vi "FocusedImageWithTrigOut.vi"() -> ()   [LabVIEW 2015]
panel:
  in  "quit remote":bool
  in  "stop sequence":bool
  in  "start sequence":bool
  in  "load sequence":bool
  in  "stop":bool
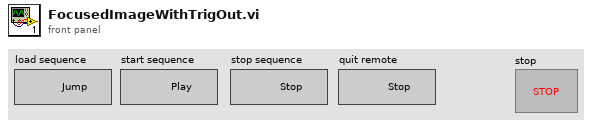
[diagram p1: front panel]
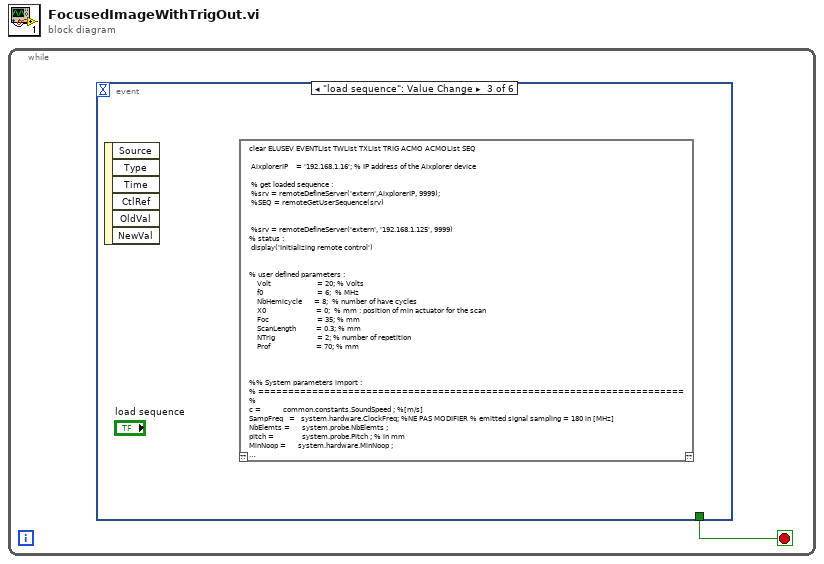
[diagram p0: block diagram]
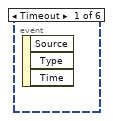
[diagram p2: hidden frame]
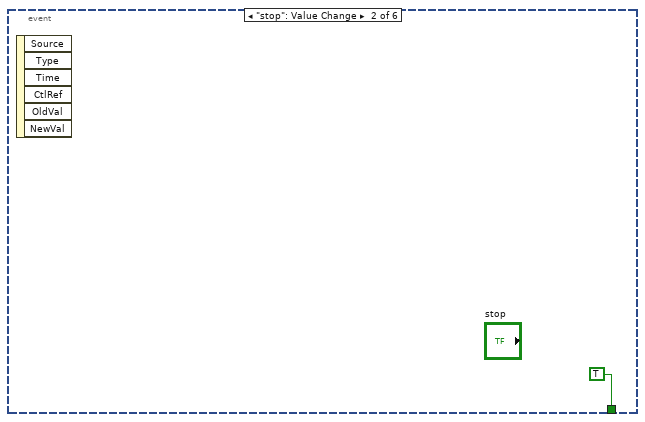
[diagram p3: hidden frame]
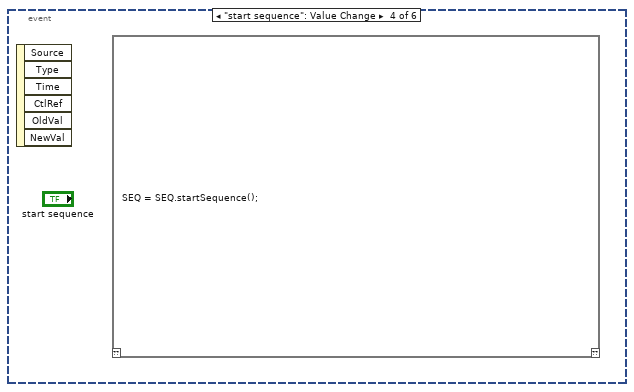
[diagram p4: hidden frame]
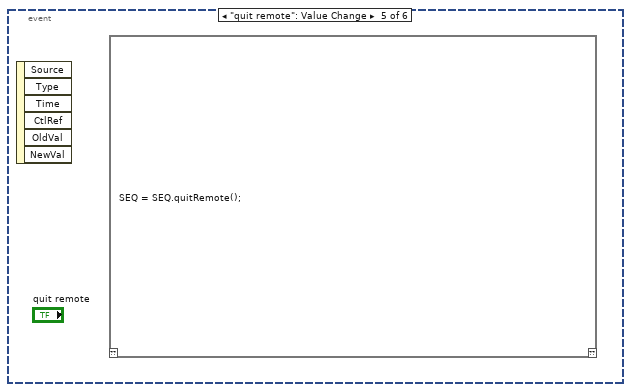
[diagram p5: hidden frame]
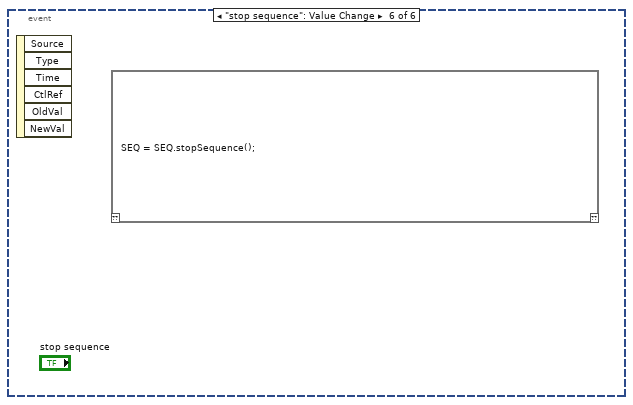
[diagram p6: hidden frame]
diagram:
  n1 = while {
    stop <- w1 stop-if-true
    n2 = event shown="[2] \"load sequence\": Value Change" {
      selector: _ -> [_ _ _ _ _ _]
      dyn-events: _ -> [_ _ _ _ _ _]
      timeout: _ -> [_ _ _ _ _ _]
      tunnel: [_ TRUE _ _ _ _] -> w1
      event Timeout {
        n3 = event-data() -> ()  [unwired: 1 in, 3 out]
      }
      event "stop": Value Change {
        n4 = event-data() -> ()  [unwired: 1 in, 6 out]
      }
      event "load sequence": Value Change {
        n5 = event-data() -> ()  [unwired: 1 in, 6 out]
        n6 = script code="clear ELUSEV EVENTList TWList TXList TRIG ACMO ACMOList SEQ\n\n AixplorerIP    = '192.168.1.16'; % IP address of the Aixplorer device\n \n % get loaded sequence :\n %srv = remoteDefineServer('extern',AixplorerIP, 9999);\n %SEQ = remoteGetUserSequence(srv)\n \n \n %srv = remoteDefineServer('extern', '192.168.1.125', 9999)\n% status :\n display('Initializing remote control')\n\n\n% user defined parameters :\n    Volt                       = 20; % Volts\n    f0                           = 6;  % MHz\n    NbHemicycle      = 8;  % number of have cycles\n    X0                         = 0;  % mm : position of min actuator for the scan\n    Foc                        = 35; % mm\n    ScanLength          = 0.3; % mm\n    NTrig                     = 2; % number of repetition\n    Prof                       = 70; % mm\n\n\n\n%% System parameters import :\n% ======================================================================= %\nc =           common.constants.SoundSpeed ; %[m/s]\nSampFreq   =   system.hardware.ClockFreq; %NE PAS MODIFIER % emitted signal sampling = 180 in [MHz]\nNbElemts =      system.probe.NbElemts ; \npitch =              system.probe.Pitch ; % in mm\nMinNoop =      system.hardware.MinNoop ;\n\n%% Focusing parameters\n% ======================================================================= %\nTxWidth       = Foc/2;           % mm : effective width for focus line\nPropagationTime = (Prof)/(c)*1e3 ; % duration for one line in \\mu s\n\n\nNoOp       = 500;             % µs minimum time between two US pulses, (5 by default ??)\nFIRBandwidth = 90;            % FIR receiving bandwidth [%] - center frequency = UF.TwFreq\nRxFreq    = 6;                % Receiving center frequency MHz , ??\n\nTrigOut    = ceil(PropagationTime);  % µs\nPause      = max( NoOp - ceil(PropagationTime) , MinNoop ); % pause duration in µs\n\n% ======================================================================= %\n%% Codage en arbitrary : delay matrix and waveform\ndt_s = 1/(SampFreq);      % unit us\npulseDuration = NbHemicycle*(0.5/f0) ; % US inital pulse duration in us\n\n\n%% Delay Law [us]\n% ======================================================================= %\n% c[m/s] -> [mm/us] ; eg factor 1e-3 in the above expression\nDelay = sqrt(Foc^2+(TxWidth/2)^2)/(c*1e-3) ...\n        - 1/(c*1e-3)*sqrt(Foc^2+((0:pitch:TxWidth)-TxWidth/2).^2);\n     \n%   figure;\n%   plot(Delay,'r')\n%   xlabel('actuator')\n%   ylabel('delays (\\mu s)')\n\n% number of steps offset dt_s for each actuators position : \n DlySmpl = round(Delay/dt_s); \n\n % common waveform for emission, square envoppe - non apodized:\n T_Wf = 0:dt_s:0.5*NbHemicycle/f0;\n Wf = sin(2*pi*f0*T_Wf); \n \n % number of time-points necessary = points in waveform + maximum delay\n % offset\n N_T = length(Wf) + max(DlySmpl); \n\n%%% construction of a delay matrix : one column / actuator\n WF_mat = zeros(N_T,length(Delay));\n\n for j = 1:length(Delay)\n     % offset for each actuator + normal waveform init\n     WF_mat(DlySmpl(j)+(1:length(Wf)),j) = Wf;\n end\n \n WF_mat_sign = sign(WF_mat); % l'aixplorer code sur 3 niveaux [-1,0,1]\n\n% figure(470);\n% imagesc((0:pitch:TxWidth)-TxWidth/2,1:N_T, WF_mat);\n% grid on\n% title('input waveform');\n% xlabel('position x');\n% ylabel('offset num ??');\n\n% ======================================================================= %\n%% Arbitrary definition of US events\n% \n% % Elusev\n\n% \n FC = remote.fc('Bandwidth', FIRBandwidth , 0);\n RX = remote.rx('fcId', 1, 'RxFreq', RxFreq, 'QFilter', 2, 'RxElemts', 0, 0);\n\n    if round((X0+ScanLength)/pitch) > NbElemts\n        warning('Scan length too long, set to maximum value');\n        ScanLength = NbElemts*pitch-X0;\n\n    end\n\nfor Nloop = 1:round(ScanLength/pitch)\n    \n    PosX     = X0 + (Nloop-1)*pitch; % center position for the line in mm\n    % EvDur = exciting pulse duration + law law + scan line duration\n    % PropagationTime , in \\mu s\n    EvtDur   = ceil( pulseDuration + max(Delay) + PropagationTime );\n\n    MedElmt  = round(PosX/pitch);\n    \n    TxElemts = MedElmt-round(TxWidth/(2*pitch)):...\n               MedElmt+floor(TxWidth/(2*pitch));\n    \n    WFtmp    = WF_mat_sign( : , ( TxElemts>0 & TxElemts<= NbElemts ) );\n    \n    %     figure(471)\n    %     imagesc(WFtmp)\n    %     drawnow\n    \n    % Flat TX\n    TXList{Nloop} = remote.tx_arbitrary('txClock180MHz', 1,'twId',Nloop,'Delays',0);\n    \n    % Arbitrary TW\n    TWList{Nloop} = remote.tw_arbitrary( ...\n        'Waveform',WFtmp', ...\n        'RepeatCH', 0, ...\n        'repeat',0 , ...\n        'repeat256', 0, ...\n        'ApodFct', 'none', ...\n        'TxElemts',TxElemts( TxElemts>0 & TxElemts <= NbElemts ), ...\n        'DutyCycle', 1, ... % duty cycle [0, 1]\n        0);\n    \n    \n    % Event\n    EVENTList{Nloop} = remote.event( ...\n        'txId', Nloop, ...\n        'rxId', 1, ...\n        'noop', Pause, ...\n        'numSamples', 128, ...\n        'skipSamples', 0, ... 128, ...\n        'duration', EvtDur, ...\n        0);\n    \nend\n\n% % ======================================================================= %\n% %% ELUSEV and ACMO definition\n% % ======================================================================= %\n\nELUSEV = elusev.elusev( ...\n    'tx',           TXList, ...\n    'tw',           TWList, ...\n    'rx',           RX,...\n    'fc',           FC,...\n    'event',        EVENTList, ...\n    'TrigOut',      TrigOut, ... 0,...\n    'TrigIn',       0,...% trigged sequence \n    'TrigAll',      0, ...% 0: sends output trigger at first emission \n    'TrigOutDelay', 0, ...\n    0);\n\nACMO = acmo.acmo( ...\n    'elusev',           ELUSEV, ...\n    'Ordering',         1, ...\n    'Repeat' ,          1, ...\n    'NbHostBuffer',     1, ...\n    'NbLocalBuffer',    1, ...\n    'ControlPts',       900, ... [900 900],...\n    'RepeatElusev',     1, ...\n    0);\n\n ACMOList{1} = ACMO;\n \n% % ======================================================================= %\n% %% Build sequence\n% % ======================================================================= %\n \n% % Probe Param\nTPC = remote.tpc( ...\n    'imgVoltage', Volt, ...\n    'imgCurrent', 1, ...% security limit for imaging current [A]\n    0);\n% \n% % USSE for the sequence\nSEQ = usse.usse( ...\n    'TPC', TPC, ...\n    'acmo', ACMOList, ...    'Loopidx',1, ...\n    'Repeat', NTrig, ...    'Popup',0, ...\n    'DropFrames', 0, ...\n    'Loop', 0, ...\n    'DataFormat', 'FF', ...\n    'Popup', 0, ...\n    0);\n\n display('Building sequence to controllor')\n \n [SEQ NbAcq] = SEQ.buildRemote();\n\n SEQ = SEQ.initializeRemote('IPaddress',AixplorerIP);\n\n\n SEQ = SEQ.loadSequence();"() -> ()  [unwired: 1 in, 1 out]
      }
      event "start sequence": Value Change {
        n7 = event-data() -> ()  [unwired: 1 in, 6 out]
        n8 = script code="SEQ = SEQ.startSequence();"() -> ()  [unwired: 1 in, 1 out]
      }
      event "quit remote": Value Change {
        n9 = event-data() -> ()  [unwired: 1 in, 6 out]
        n10 = script code="SEQ = SEQ.quitRemote();"() -> ()  [unwired: 1 in, 1 out]
      }
      event "stop sequence": Value Change {
        n11 = event-data() -> ()  [unwired: 1 in, 6 out]
        n12 = script code="SEQ = SEQ.stopSequence();"() -> ()  [unwired: 1 in, 1 out]
      }
    }
  }
